vi "Video feed info class VI - change video info.vi"(0 "Video feed info in":refnum<class "Video feed info.lvclass">, 1 "Avi Refnum (duplicate)":T1, 2 "file path":path, 5 "Image Type":T2 items=["Grayscale (U8)", "Grayscale (I16)", "Grayscale (SGL)", "Complex (CSG)", "RGB (U32)", "HSL (U32)", "RGB (U64)", "Grayscale (U16)"], 7 "width":u32, 9 "height":u32, 11 "error in (no error)":errorcluster, 12 "FPS":u32, 13 "Number of Frames":u32) -> (4 "Video feed info out":refnum<class "Video feed info.lvclass">, 15 "error out":errorcluster)   [LabVIEW 2010, in "Video feed info.lvclass"]
uses:
  Video feed info.lvclass
  <vilib>/vision/Avi1.llb/AviRefnum.ctl
  Video feed info.lvclass/Video feed info.ctl
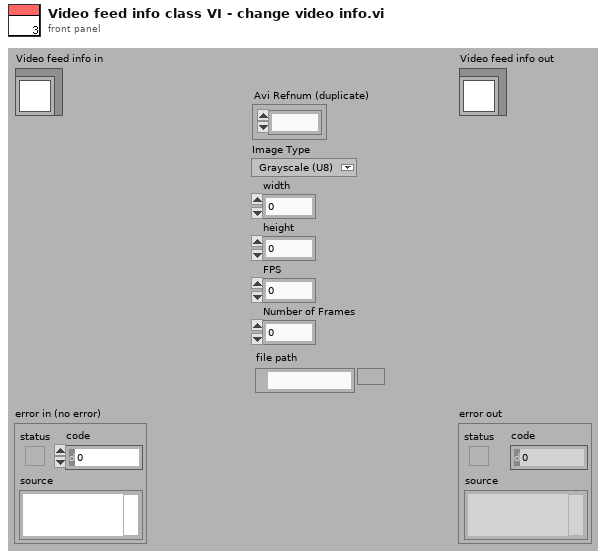
[diagram p1: front panel]
types:
  T1 = typedef "AviRefnum.ctl" = refnum<k1>
  T2 = typedef "Image Type" = u32
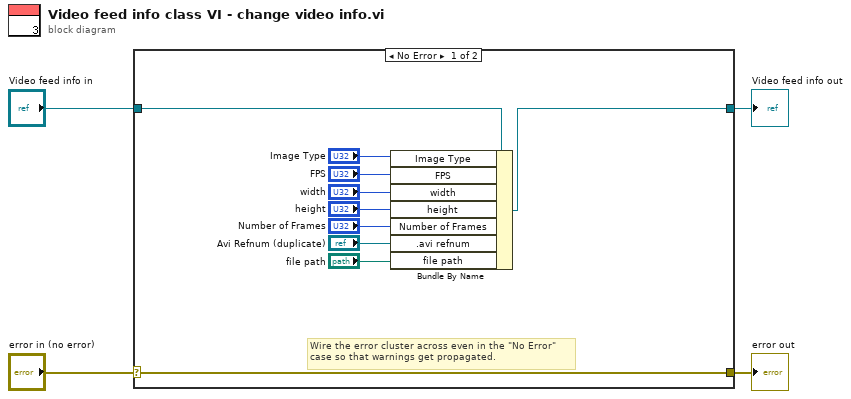
[diagram p0: block diagram]
diagram:
  n1 = case shown="No Error" "error in (no error)" {
    selector: "error in (no error)" -> [w14 w16]
    tunnel: [w14 w16] -> w3
    tunnel: [w12 w15] -> w1
    tunnel: "Video feed info in" -> [w13 w15]
    frame No Error {
      # "Wire the error cluster across even in the \"No Error\"\ncase so that warnings get propagated."
      n2 = Bundle By Name(cluster=w13, "Image Type"="Image Type", "FPS"="FPS", "width"="width", "height"="height", "Number of Frames"="Number of Frames", ".avi refnum"="Avi Refnum (duplicate)", "file path"="file path") -> (w12:refnum<class "Video feed info.lvclass">)
    }
    frame Error {
    }
  }
  "error out" <- w3
  "Video feed info out" <- w1
